vi "DataCluster.vi"() -> ()   [LabVIEW 2019]
uses:
  Data Cluster.ctl
  <vilib>/vision/Image Controls.llb/IMAQ Image.ctl
panel:
  in  "Data Cluster":T1
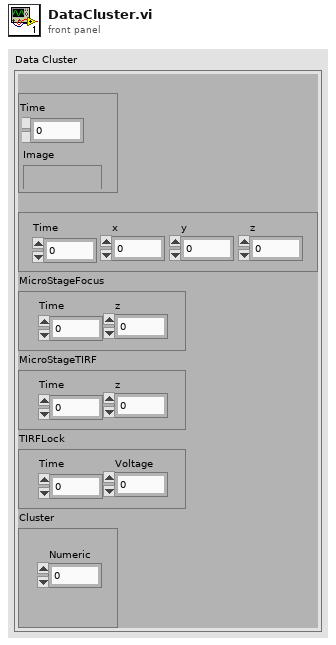
[diagram p1: front panel]
types:
  T1 = typedef "Data Cluster.ctl" = cluster{"RawImage":cluster{"Time":dbl, "Image":T2}, "NanoStage":cluster{"x":dbl, "y":dbl, "z":dbl, "Time":dbl}, "MicroStageFocus":cluster{"Time":dbl, "z":dbl}, "MicroStageTIRF":cluster{"Time":dbl, "z":dbl}, "TIRFLock":cluster{"Time":dbl, "Voltage":dbl}, "Cluster":cluster{"Numeric":dbl}}
  T2 = typedef "IMAQ Image.ctl" = refnum<image>
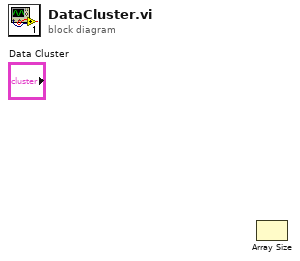
[diagram p0: block diagram]
diagram:
  n1 = Array Size() -> (array=w1:dbl[])  [unwired: 1 out]
